vi "Drop Message Core.vi"(11 "Measure Msg in":refnum<class "Measure Msg.lvclass">) -> ()   [LabVIEW 2013, in "Universal Power Meter.lvlib" / "Measure Msg.lvclass"]
doc: "(<B>Filename</B>: Actor Framework.lvlib:Message.lvclass:Drop Message Core.vi)\n\nDefines what a message does if it is in the message queue when the queue is released. At this point, the actor has shut down, so it will never process the message.\n\nBy default, this method does nothing. A child class may override it to define behavior. National Instruments provides the Reply Msg class to override this method. This class releases its internal queue, which causes any caller of the Send Message and Wait For Response method to stop waiting and return an error."
uses:
  Measure Msg.lvclass
  <vilib>/ActorFramework/Message/Message.lvclass
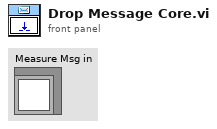
[diagram p1: front panel]
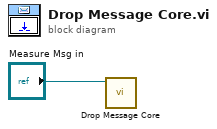
[diagram p0: block diagram]
diagram:
  n1 = call-parent "Drop Message Core.vi"("Message in"="Measure Msg in") -> ()  [unwired: 11 in]
